vi "String Length.vi"() -> ()   [LabVIEW 2020]
doc: "This example shows how String Length function operates with different data types."
panel:
  in  "Tab Control":T1(tab)
  out "Length":i32
  in  "String":string="To"
  out "Array of Lengths":i32[](array[numeric])
  in  "Array of Strings":string[](array[string])=["Array", "Of", "Strings"]
  out "Cluster of Lengths":T2
  in  "Cluster of Strings":T3={"String"="string one", "String 2"="string two", "String 3"="string three"}
  out "Lengths":cluster{"Lengths":i32[], "Length":i32}
  in  "Cluster":cluster{"Array":string[], "String":string}={"Array"=["array", "in", "cluster"], "String"="string in cluster"}
  out "Array of Lengths":cluster{"Length":i32, "Length 2":i32}[](array[cluster])
  in  "Array of Clusters":cluster{"String":string, "String 2":string}[](array[cluster])=[{"String"="array", "String 2"="of"}, {"String"="clusters", "String 2"=""}]
  # "Overview: Demonstrates how the String Length function operates with different data types.\nInstructions:\n1. Run the VI.\n2. Examine the different cases."
  # "The most common use of the String Length function is to calculate the length of a single string."
  # "When an array of strings is wired to the String Length function, the length of each string is calculated and returned as an array."
  # "When a cluster of strings is wired to the String Length function, the length of each string is calculated and returned as a cluster of lengths."
  # "When a cluster of arrays of strings and scalar strings is wired to the String Length function, the lengths of all strings are calculated and returned in a corresponding cluster containing arrays of lengths and scalar lengths appropriately."
  # "When an array of clusters is wired to the String Length function, the lengths of all strings are calculated and returned in a corresponding array of clusters of lengths."
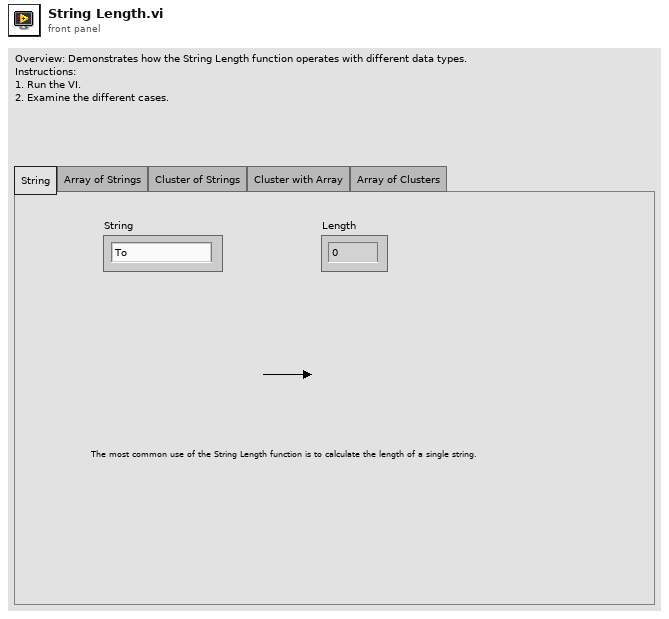
[diagram p1: front panel]
types:
  T1 = enum32{"String", "Array of Strings", "Cluster of Strings", "Cluster with Array", "Array of Clusters"}
  T2 = cluster{"Length":i32, "Length 2":i32, "Length 3":i32}
  T3 = cluster{"String":string, "String 2":string, "String 3":string}
  T4 = cluster{"String":i32, "String 2":i32, "String 3":i32}
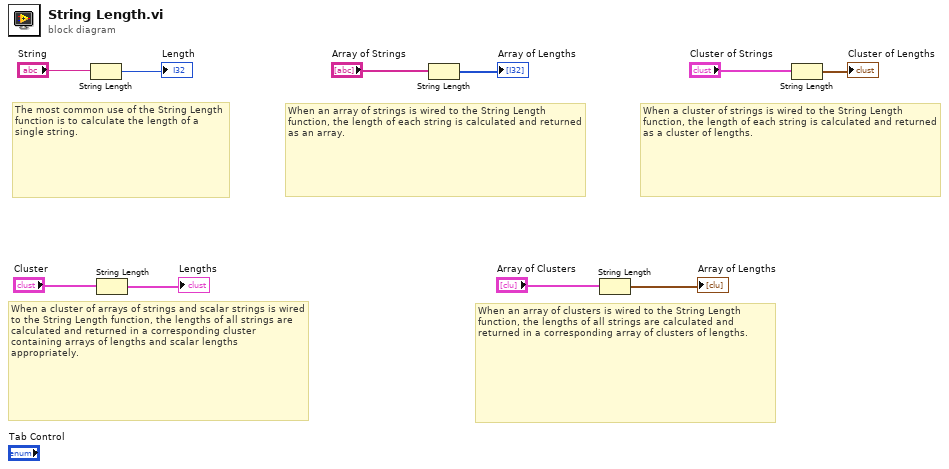
[diagram p0: block diagram]
diagram:
  # "When an array of clusters is wired to the String Length function, the lengths of all strings are calculated and returned in a corresponding array of clusters of lengths."
  # "When a cluster of arrays of strings and scalar strings is wired to the String Length function, the lengths of all strings are calculated and returned in a corresponding cluster containing arrays of lengths and scalar lengths appropriately."
  # "When a cluster of strings is wired to the String Length function, the length of each string is calculated and returned as a cluster of lengths."
  # "When an array of strings is wired to the String Length function, the length of each string is calculated and returned as an array."
  # "The most common use of the String Length function is to calculate the length of a single string."
  n1 = String Length(string="String") -> (length=→"Length":i32)
  n2 = String Length(string="Cluster") -> (length=→"Lengths":cluster{"Array":i32[], "String":i32})
  n3 = String Length(string="Array of Strings") -> (length=→"Array of Lengths":i32[])
  n4 = String Length(string="Array of Clusters") -> (length=→"Array of Lengths":cluster{"String":i32, "String 2":i32}[])
  n5 = String Length(string="Cluster of Strings") -> (length=→"Cluster of Lengths":T4)
